vi "FTP_PASV.vi"(0 "connection ID":refnum<k5>, 2 "error in":errorcluster) -> (3 "connection ID out":refnum<k5>, 4 "Passive Port":T1, 5 "Good Reply?":bool, 6 "error out":errorcluster)   [LabVIEW 2012]
panel:
  out "reply string":string
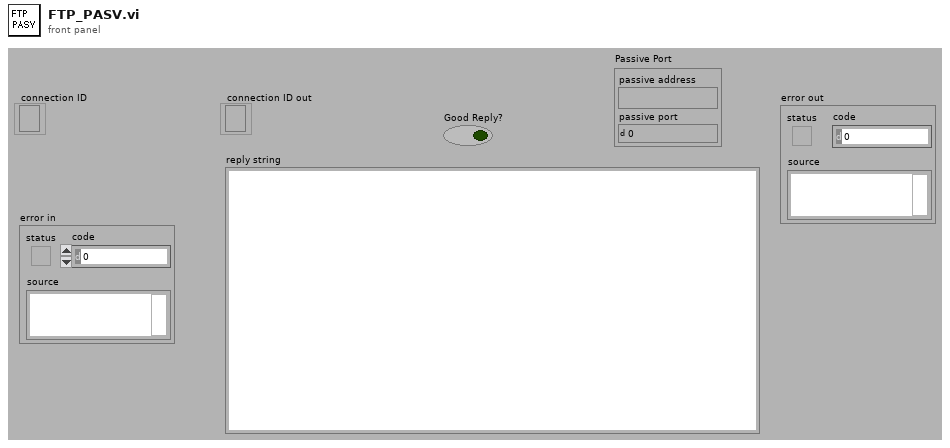
[diagram p1: front panel]
types:
  T1 = cluster{"passive address":string, "passive port":u16}
  T2 = enum16{"unknown", "100 + Prelim", "200 + ", "300 + Intermed", "400 - Transient", "500 - Permanent"}
  T3 = cluster{"[u8][0]":u8, "[u8][1]":u8, "[u8][2]":u8, "[u8][3]":u8, "[u8][4]":u8, "[u8][5]":u8}
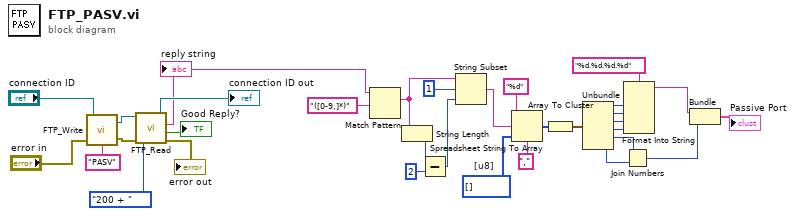
[diagram p0: block diagram]
diagram:
  w17 = u8[] []  # [u8]
  n1 = call <userlib>:"FTP_Write.vi"("Cmd"="PASV", "error in"="error in", "connection ID in"="connection ID") -> ("error out"=w25:errorcluster, "connection ID out"=w26:refnum<k5>)  [unwired: 1 in]
  n2 = call <userlib>:"FTP_Read.vi"("error In"=w25, "expected class"=T2."200 + ", "connection ID"=w26) -> ("error out"=→"error out":errorcluster, "Good Reply?"=→"Good Reply?":bool, "reply string"=w5:string, "connection ID out"=→"connection ID out":refnum<k5>)  [unwired: 1 out]
  "reply string" <- w5
  n3 = Match Pattern(string=w5, regular expression="([0-9,]*)") -> (match substring=w23:string)  [unwired: 4 out]
  n4 = String Length(string=w23) -> (length=w22:i32)
  n5 = Subtract(x=w22, y=2) -> (x-y=w7:i32)
  n6 = String Subset(string=w23, offset (0)=1 ("length"), length (rest)=w7) -> (substring=w20:string)
  n7 = Spreadsheet String To Array(delimiter (Tab)=",", format string="%d", spreadsheet string=w20, array type (2D Dbl)=w17) -> (array=w16:u8[])
  n8 = Array To Cluster(array=w16) -> (cluster=w15:T3)
  n9 = Unbundle(w15) -> ("[u8][0]"=w8:u8, "[u8][1]"=w9:u8, "[u8][2]"=w10:u8, "[u8][3]"=w11:u8, "[u8][4]"=w14:u8, "[u8][5]"=w13:u8)
  n10 = Join Numbers(hi=w14, lo=w13) -> ((hi.lo)=w3:u16)
  n11 = Format Into String(format string="%d.%d.%d.%d", w8, w9, w10, w11) -> (resulting string=w4:string)  [unwired: 2 in, 1 out]
  n12 = Bundle(w4, w3) -> (→"Passive Port":cluster{string, u16})  [unwired: 1 out]
